vi "FR Read settings from file.vi"(8 "error in (passthrough)":errorcluster) -> (0 "error out":errorcluster, 3 "FFmeter settings":T1={"AC Source"={"AC Source type"=enum."Fluke 5XXX calibrator", "VISA"="", "Ref. clock (Hz)"=0.0, "status ref"=refnum}, "TWM pipe"="\\\\.\\pipe\\TWM:server", "Measurement status ref"=refnum, "TWM Status ref"=refnum, "Abort ref"=refnum, "DC meter"={"DC meter type"=enum."H/A/K 3458", "DC meter VISA"="", "NPLC"=10, "status ref"=refnum}, "Measurement properties"={"Measurement frequencies (Hz)"=[1000.0], "Sampling frequency (Hz)"=500000.0, "Signal amplitude (V)"=4.5, "AC-DC settle time (s)"=20.0, "Record length (multiples of period)"=[1000.0, 10000.0, 1000.0], "Measurement template file"=path "", "Row of START keyword"=1, "Row of STOP keyword"=0, "Calculate RMS from samples"=FALSE, "AC-DC warm up time (s)"=300.0, "Measurement template line"=[], "DC meter readings No."=10, "Algorithm"="TWM-WFFT"}, "Skip waiting ref"=refnum, "Octave paths"={"GNU Octave path"=path "C:/Program Files/GNU Octave/Octave-6.2.0/mingw64/bin", "TWM+QWTB path"=path "C:/Users/labina/Desktop/TWM-1.8.7.0-full/octprog", "lvlib path"=path "D:/martin/WAC/WACsw - github/control_software/Filter function meter/external libraries/GOLPI 0.7.3.1 source distribution LV 20.0 32 bit/lv_proc.dll"}, "Template definition"={"Keywords column"=0, "Sig. freq. column"=1, "Rec. len. column"=2, "Meas. points. row min to read"=9, "Meas. points. row max to read"=1509, "Properties column"=4, "Properties row start"=1, "Properties row end"=5, "Keyword START regexp"="", "Keyword STOP regexp"="", "HW data column"=7, "HW data row start"=1, "HW data row end"=3, "TIme and date column start"=3, "Digitizer value column start "=4, "DC mean column start "=6, "DC readings column start"=10}} {"Measurement properties"."Record length (multiples of period)" format="%#_3p"; "Measurement properties"."Sampling frequency (Hz)" format="%#_3p"; "Measurement properties"."Measurement frequencies (Hz)" format="%#_3p"})   [LabVIEW 2020]
uses:
  FR GUI/Type definitions/FFmeter settings.ctl
  General AC source/Type definitions/AC Source.ctl
  General AC source/Type definitions/AC Source type.ctl
  General DC meter/Type definitions/DC meter.ctl
  General DC meter/Type definitions/DC meter type.ctl
  FR Measurement/Type definitions/FR Measuement properties.ctl
  Type definitions/FR Template definition.ctl
  <vilib>/Utility/xml.llb/Read From XML File(string).vi
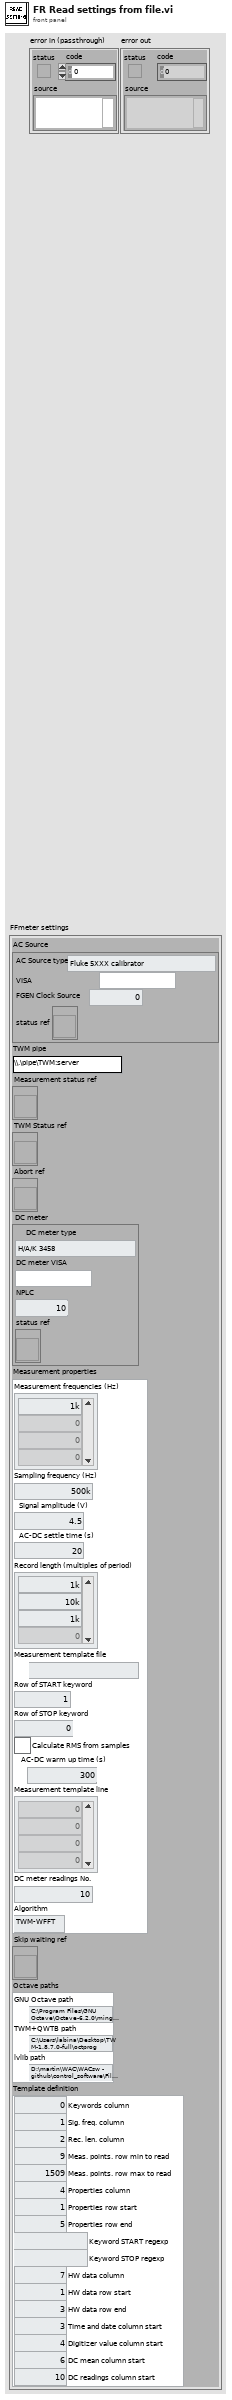
[diagram p1: front panel]
types:
  T1 = typedef "FFmeter settings.ctl" = cluster{"AC Source":T2, "TWM pipe":string, "Measurement status ref":refnum<vi>, "TWM Status ref":refnum<vi>, "Abort ref":refnum<vi>, "DC meter":T4, "Measurement properties":T6, "Skip waiting ref":refnum<vi>, "Octave paths":cluster{"GNU Octave path":path, "TWM+QWTB path":path, "lvlib path":path}, "Template definition":T7}
  T2 = typedef "AC Source.ctl" = cluster{"AC Source type":T3, "VISA":refnum<visa-resource-name>, "Ref. clock (Hz)":dbl, "status ref":refnum<vi>}
  T3 = typedef "AC Source type.ctl" = enum16{"Fluke 5XXX calibrator", "Tektronix AFG3000 series", "dummy"}
  T4 = typedef "DC meter.ctl" = cluster{"DC meter type":T5, "DC meter VISA":refnum<visa-resource-name>, "NPLC":i32, "status ref":refnum<vi>}
  T5 = typedef "DC meter type.ctl" = enum16{"H/A/K 3458", "FLuke 8508A", "dummy"}
  T6 = typedef "FR Measuement properties.ctl" = cluster{"Measurement frequencies (Hz)":dbl[], "Sampling frequency (Hz)":dbl, "Signal amplitude (V)":dbl, "AC-DC settle time (s)":dbl, "Record length (multiples of period)":dbl[], "Measurement template file":path, "Row of START keyword":i32, "Row of STOP keyword":i32, "Calculate RMS from samples":bool, "AC-DC warm up time (s)":dbl, "Measurement template line":i32[], "DC meter readings No.":i32, "Algorithm":string}
  T7 = typedef "FR Template definition.ctl" = cluster{"Keywords column":i32, "Sig. freq. column":i32, "Rec. len. column":i32, "Meas. points. row min to read":i32, "Meas. points. row max to read":i32, "Properties column":i32, "Properties row start":i32, "Properties row end":i32, "Keyword START regexp":string, "Keyword STOP regexp":string, "HW data column":i32, "HW data row start":i32, "HW data row end":i32, "TIme and date column start":i32, "Digitizer value column start ":i32, "DC mean column start ":i32, "DC readings column start":i32}
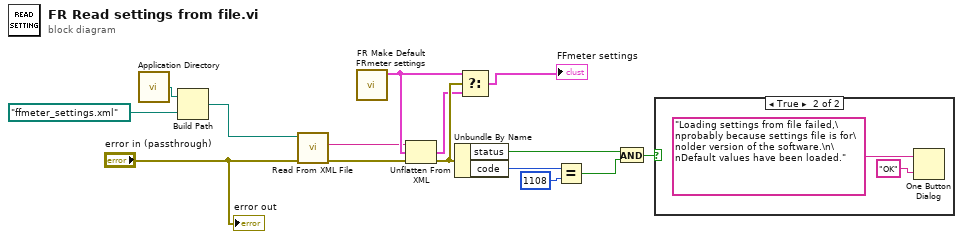
[diagram p0: block diagram]
diagram:
  n1 = call <vilib>:"Application Directory.vi"() -> ("Application Directory"=w14:path)
  n2 = Build Path(base path=w14, name or relative path=path "ffmeter_settings.xml") -> (appended path=w12:path)
  n3 = call-poly <vilib>:"Read From XML File.vi"("error in (no error)"="error in (passthrough)", "XML File Path"=w12) -> ("error out"=w10:errorcluster, "XML Elements"=w11:string)  [unwired: 7 in, 1 out]
  n4 = call "FR Make Default FRmeter settings.vi"() -> ("FFmeter settings"=w15:T1)  [unwired: 11 in]
  n5 = Unflatten From XML(xml string=w11, type=w15, error in (no error)=w10) -> (value=w3:T1, error out=w4:errorcluster)
  n6 = Unbundle By Name(w4) -> ("status"=w6:bool, "code"=w9:i32)
  n7 = Select(t=w15, s=w4, f=w3) -> (s? t:f=→"FFmeter settings":T1)
  n8 = Equal?(x=w9, y=1108) -> (x = y?=w7:bool)
  n9 = And(x=w6, y=w7) -> (x .and. y?=w5:bool)
  n10 = case shown="True" w5 {
    frame False {
    }
    frame True {
      n11 = One Button Dialog(message="Loading settings from file failed,\nprobably because settings file is for\nolder version of the software.\n\nDefault values have been loaded.", button name ("OK")="OK") -> ()  [unwired: 1 out]
    }
  }
  "error out" <- "error in (passthrough)"
